vi "AccelGyro constants Read-Write, standalone.vi"() -> ()   [LabVIEW 2015]
uses:
  Ctls/AccelGyro constants.ctl
panel:
  in  "AccelGyro constants out":T1={"gyrRange"=125.0, "accRange"=2.0, "gx offset"=0.0, "gy offset"=0.0, "gz offset"=0.0, "ax offset"=0.0, "ay offset"=0.0, "az offset"=0.0, "axyz scale"=1.0}
  out "AccelGyro constants returned":T1={"gyrRange"=125.0, "accRange"=2.0, "gx offset"=0.0, "gy offset"=0.0, "gz offset"=0.0, "ax offset"=0.0, "ay offset"=0.0, "az offset"=0.0, "axyz scale"=1.0}
  in  "Error In":errorcluster
  out "ACK ok":bool
  in  "VISA resource name in":refnum<visa-resource-name>
  out "Error out":errorcluster
  in  "R / W":string(combo)="R"
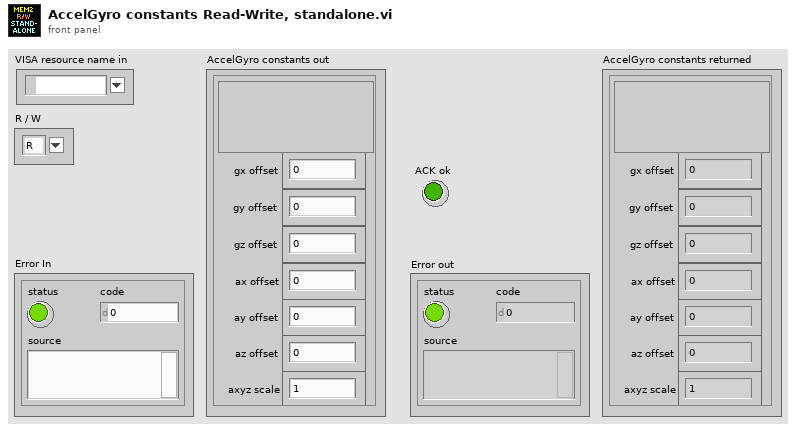
[diagram p1: front panel]
types:
  T1 = typedef "AccelGyro constants.ctl" = cluster{"gyrRange":sgl, "accRange":sgl, "gx offset":sgl, "gy offset":sgl, "gz offset":sgl, "ax offset":sgl, "ay offset":sgl, "az offset":sgl, "axyz scale":sgl}
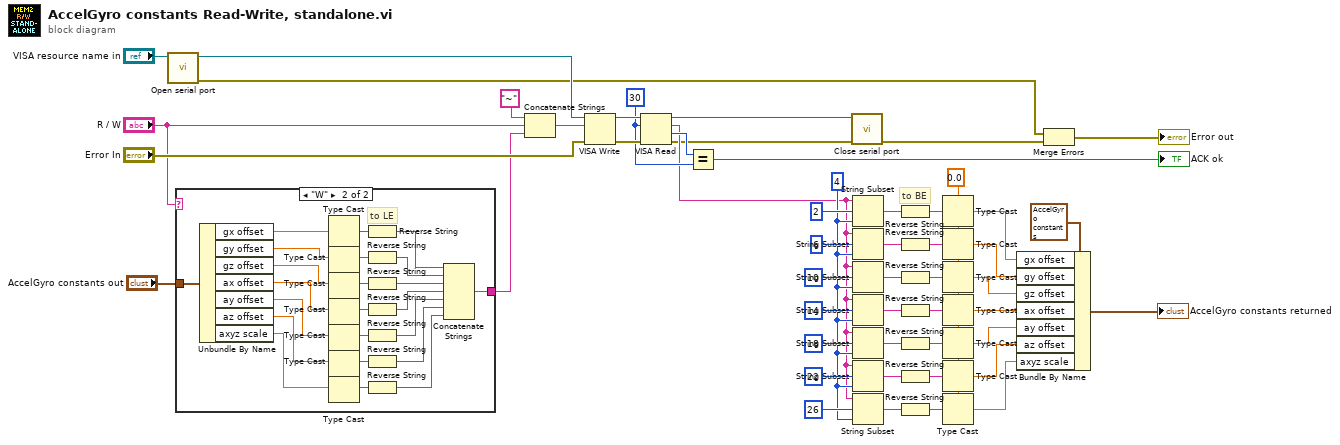
[diagram p0: block diagram]
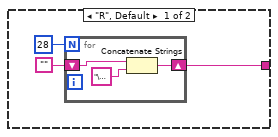
[diagram p2: hidden frame]
diagram:
  w22 = 4 ("length (rest)")
  w20 = sgl 0.0
  w44 = u32 30 ("byte count")
  # "to BE"
  n1 = call "Open serial port.vi"("VISA resource name"="VISA resource name in") -> ("Error out"=w38:errorcluster, "VISA resource name out"=w40:refnum<visa-resource-name>)  [unwired: 9 in]
  n2 = case shown="\"W\"" "R / W" {
    tunnel: "AccelGyro constants out" -> [_ w80]
    tunnel: [w53 w72] -> w42
    frame "R", Default {
      n3 = for {
        N: 28 -> [_]
        shift-right: [w56] -> w53
        shift-left: "" -> [w55]
        n4 = Concatenate Strings(w55, "\u0000") -> (w56:string)
      }
    }
    frame "W" {
      # "to LE"
      n5 = Unbundle By Name(w80) -> ("gx offset"=w79:sgl, "gy offset"=w78:sgl, "gz offset"=w77:sgl, "ax offset"=w76:sgl, "ay offset"=w75:sgl, "az offset"=w74:sgl, "axyz scale"=w73:sgl)
      n6 = Type Cast(x=w79) -> (*(type *) &x=w71:string)  [unwired: 1 in]
      n7 = Type Cast(x=w78) -> (*(type *) &x=w70:string)  [unwired: 1 in]
      n8 = Type Cast(x=w77) -> (*(type *) &x=w69:string)  [unwired: 1 in]
      n9 = Type Cast(x=w76) -> (*(type *) &x=w68:string)  [unwired: 1 in]
      n10 = Type Cast(x=w75) -> (*(type *) &x=w67:string)  [unwired: 1 in]
      n11 = Type Cast(x=w74) -> (*(type *) &x=w66:string)  [unwired: 1 in]
      n12 = Type Cast(x=w73) -> (*(type *) &x=w65:string)  [unwired: 1 in]
      n13 = Reverse String(1:w71) -> (0:w64:string)
      n14 = Reverse String(1:w70) -> (0:w63:string)
      n15 = Reverse String(1:w69) -> (0:w62:string)
      n16 = Reverse String(1:w68) -> (0:w61:string)
      n17 = Reverse String(1:w67) -> (0:w60:string)
      n18 = Reverse String(1:w66) -> (0:w59:string)
      n19 = Reverse String(1:w65) -> (0:w58:string)
      n20 = Concatenate Strings(w64, w63, w62, w61, w60, w59, w58) -> (w72:string)
    }
  }
  n21 = Concatenate Strings("~" ("string"), "R / W", w42) -> (w46:string)
  n22 = VISA Write(VISA resource name=w40, write buffer=w46, error in (no error)="Error In") -> (VISA resource name out=w50:refnum<visa-resource-name>, error out=w49:errorcluster)  [unwired: 1 out]
  n23 = VISA Read(VISA resource name=w50, byte count=w44, error in (no error)=w49) -> (VISA resource name out=w39:refnum<visa-resource-name>, read buffer=w21:string, return count=w45:u32, error out=w17:errorcluster)
  n24 = Equal?(x=w45, y=w44) -> (x = y?=→"ACK ok":bool)
  n25 = call "Close serial port.vi"("Error in"=w17, "VISA resource name"=w39) -> ("Error out"=w16:errorcluster)  [unwired: 9 in]
  n26 = String Subset(string=w21, offset (0)=2 ("length (rest)"), length (rest)=w22) -> (substring=w14:string)
  n27 = String Subset(string=w21, offset (0)=6 ("length (rest)"), length (rest)=w22) -> (substring=w12:string)
  n28 = String Subset(string=w21, offset (0)=10 ("length (rest)"), length (rest)=w22) -> (substring=w10:string)
  n29 = String Subset(string=w21, offset (0)=14 ("length (rest)"), length (rest)=w22) -> (substring=w9:string)
  n30 = String Subset(string=w21, offset (0)=18 ("length (rest)"), length (rest)=w22) -> (substring=w8:string)
  n31 = String Subset(string=w21, offset (0)=22 ("length (rest)"), length (rest)=w22) -> (substring=w7:string)
  n32 = String Subset(string=w21, offset (0)=26 ("length (rest)"), length (rest)=w22) -> (substring=w6:string)
  n33 = Reverse String(1:w14) -> (0:w13:string)
  n34 = Reverse String(1:w12) -> (0:w11:string)
  n35 = Reverse String(1:w10) -> (0:w2:string)
  n36 = Reverse String(1:w9) -> (0:w3:string)
  n37 = Reverse String(1:w8) -> (0:w4:string)
  n38 = Reverse String(1:w7) -> (0:w1:string)
  n39 = Reverse String(1:w6) -> (0:w5:string)
  n40 = Type Cast(type=w20, x=w13) -> (*(type *) &x=w35:sgl)
  n41 = Type Cast(type=w20, x=w11) -> (*(type *) &x=w34:sgl)
  n42 = Type Cast(type=w20, x=w2) -> (*(type *) &x=w33:sgl)
  n43 = Type Cast(type=w20, x=w3) -> (*(type *) &x=w32:sgl)
  n44 = Type Cast(type=w20, x=w4) -> (*(type *) &x=w31:sgl)
  n45 = Type Cast(type=w20, x=w1) -> (*(type *) &x=w19:sgl)
  n46 = Type Cast(type=w20, x=w5) -> (*(type *) &x=w18:sgl)
  n47 = Bundle By Name(cluster=T1 {"gyrRange"=0.0, "accRange"=0.0, "gx offset"=0.0, "gy offset"=0.0, "gz offset"=0.0, "ax offset"=0.0, "ay offset"=0.0, "az offset"=0.0, "axyz scale"=1.0} ("AccelGyro constants"), "gx offset"=w35, "gy offset"=w34, "gz offset"=w33, "ax offset"=w32, "ay offset"=w31, "az offset"=w19, "axyz scale"=w18) -> (→"AccelGyro constants returned":T1)
  n48 = Merge Errors(w38, w16) -> (→"Error out":errorcluster)
